vi "Para_ERD_Fxxx.vi"(7 "GEA Inputs":T4={"Source"=228, "Destination"=36} {"Destination" format="%.0x"; "Source" format="%.0x"}, 8 "Error In":errorcluster, 10 "Read ERD List":T2[](array[typedef])=[{"ERD Number"=62976, "Data Type"=enum."string"}, {"ERD Number"=62977, "Data Type"=enum."string"}, {"ERD Number"=63015, "Data Type"=enum."string"}, {"ERD Number"=63016, "Data Type"=enum."string"}, {"ERD Number"=63017, "Data Type"=enum."string"}, {"ERD Number"=63018, "Data Type"=enum."string"}, {"ERD Number"=63019, "Data Type"=enum."string"}, {"ERD Number"=63020, "Data Type"=enum."string"}, {"ERD Number"=63021, "Data Type"=enum."string"}, {"ERD Number"=63022, "Data Type"=enum."string"}, {"ERD Number"=63023, "Data Type"=enum."string"}, {"ERD Number"=63024, "Data Type"=enum."string"}, {"ERD Number"=63025, "Data Type"=enum."string"}, {"ERD Number"=63026, "Data Type"=enum."string"}, {"ERD Number"=63028, "Data Type"=enum."string"}, {"ERD Number"=63029, "Data Type"=enum."string"}, {"ERD Number"=63030, "Data Type"=enum."string"}, {"ERD Number"=63031, "Data Type"=enum."string"}, {"ERD Number"=63032, "Data Type"=enum."string"}, {"ERD Number"=63033, "Data Type"=enum."string"}, {"ERD Number"=63034, "Data Type"=enum."string"}, {"ERD Number"=63035, "Data Type"=enum."string"}, {"ERD Number"=63036, "Data Type"=enum."string"}, {"ERD Number"=63037, "Data Type"=enum."string"}, {"ERD Number"=63038, "Data Type"=enum."string"}, {"ERD Number"=63039, "Data Type"=enum."string"}, {"ERD Number"=63040, "Data Type"=enum."string"}, {"ERD Number"=63041, "Data Type"=enum."string"}, {"ERD Number"=63042, "Data Type"=enum."string"}, {"ERD Number"=63043, "Data Type"=enum."string"}, {"ERD Number"=63044, "Data Type"=enum."string"}, {"ERD Number"=63045, "Data Type"=enum."string"}, {"ERD Number"=63046, "Data Type"=enum."string"}, {"ERD Number"=63047, "Data Type"=enum."string"}, {"ERD Number"=63048, "Data Type"=enum."string"}, {"ERD Number"=63049, "Data Type"=enum."string"}, {"ERD Number"=63050, "Data Type"=enum."string"}, {"ERD Number"=63052, "Data Type"=enum."string"}, {"ERD Number"=63053, "Data Type"=enum."string"}, {"ERD Number"=63054, "Data Type"=enum."string"}, {"ERD Number"=63055, "Data Type"=enum."string"}, {"ERD Number"=63056, "Data Type"=enum."string"}, {"ERD Number"=63060, "Data Type"=enum."string"}, {"ERD Number"=63061, "Data Type"=enum."string"}, {"ERD Number"=63067, "Data Type"=enum."string"}, {"ERD Number"=63068, "Data Type"=enum."string"}, {"ERD Number"=63072, "Data Type"=enum."string"}, {"ERD Number"=63073, "Data Type"=enum."string"}, {"ERD Number"=63074, "Data Type"=enum."string"}, {"ERD Number"=63075, "Data Type"=enum."string"}, {"ERD Number"=63076, "Data Type"=enum."string"}, {"ERD Number"=63077, "Data Type"=enum."string"}, {"ERD Number"=63078, "Data Type"=enum."string"}, {"ERD Number"=63079, "Data Type"=enum."string"}, {"ERD Number"=63080, "Data Type"=enum."string"}, {"ERD Number"=63081, "Data Type"=enum."string"}] {"ERD Number" format="%.0x"}, 11 "GEA2 Reference In":refnum<k24>) -> (0 "Error Out":errorcluster, 1 "ERD Data Out":T3[](array[typedef]) {"ERD Number" format="%.0x"}, 2 "F6XX":T1, 3 "GEA2 Reference Out":refnum<k24>)   [LabVIEW 2023]
uses:
  type defs/F6_ERD_Control.ctl
  Common/LabVIEW GEA2 Toolkit/GEA3/type defs/Source_Destination.ctl
  D:/Common/LabVIEW GEA2 Toolkit/source/GEA3 DLL Source/GeaCommunication.dll
  Common/LabVIEW GEA2 Toolkit/source/GEA3 DLL Source/GeaCommunication.dll
  Common/LabVIEW GEA2 Toolkit/GEA3/type defs/ERD Read Data Out.ctl
  Common/LabVIEW GEA2 Toolkit/GEA3/type defs/ERD Read Data In.ctl
panel:
  out "number":u32
  in  "F6XX 2":T1
  in  "F6XX":T1
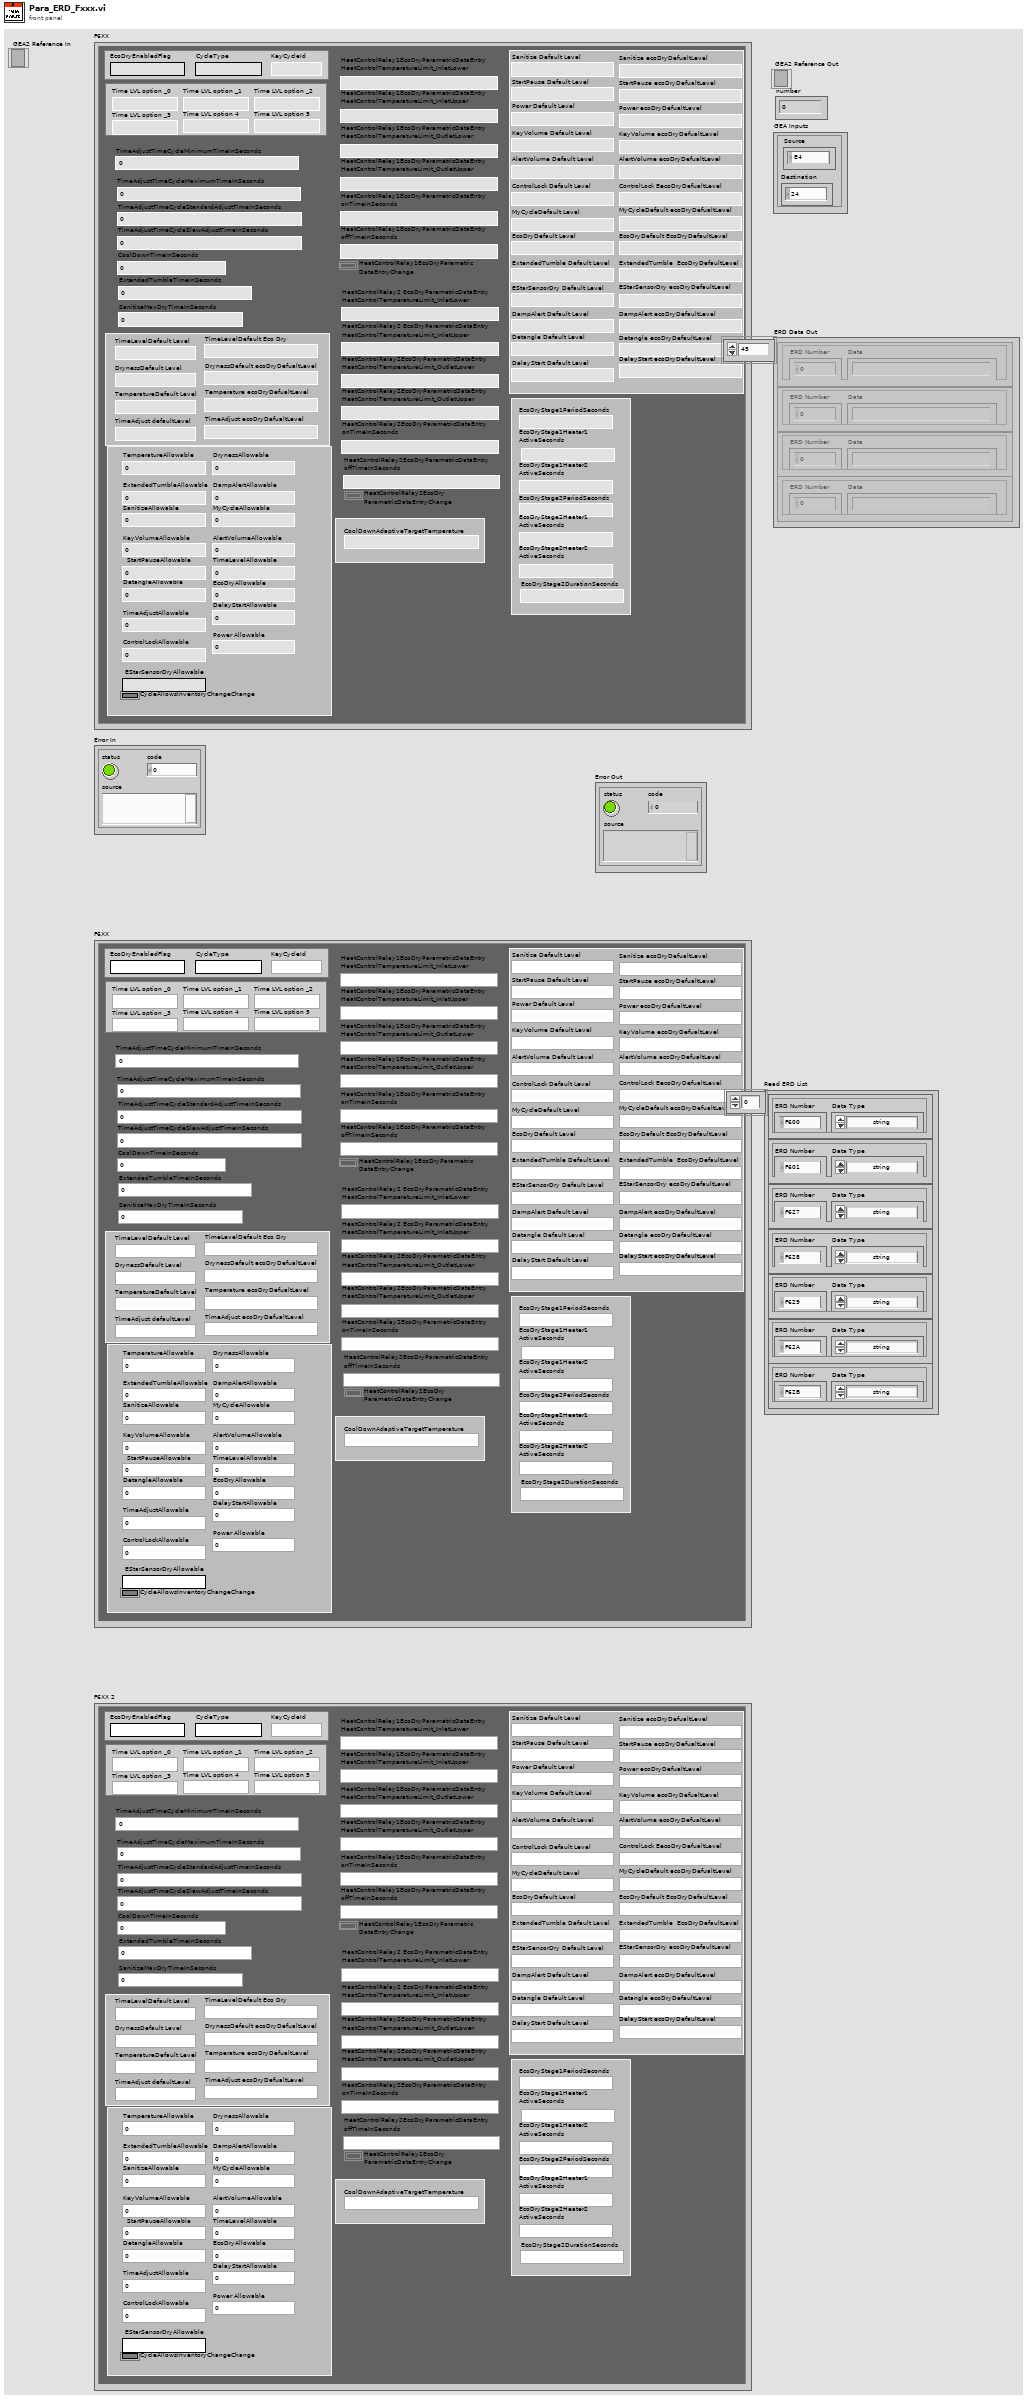
[diagram p1: front panel]
types:
  T1 = typedef "F6_ERD_Control.ctl" = cluster{"EcoDryEnabledFlag":string, "KeyCycleId":u8, "CycleType":string, "Time LVL option 5":u32, "Time LVL option 4":u32, "Time LVL option _3":u32, "Time LVL option _2":u32, "Time LVL option _1":u32, "Time LVL option _0":u32, "CoolDownTimeInSeconds":u32, "TimeAdjustTimeCycleMinimumTimeInSeconds":u32, "TimeAdjustTimeCycleMaximumTimeInSeconds":u32, "TimeAdjustTimeCycleStandardAdjustTimeInSeconds":u32, "TimeAdjustTimeCycleSlewAdjustTimeInSeconds":u32, "ExtendedTumbleTimeInSeconds":u32, "SanitizeMaxDryTimeInSeconds":u32, "TemperatureDefault Level":u8, "Temperature ecoDryDefualtLevel":u8, "DrynessDefault Level":u8, "DrynessDefault ecoDryDefualtLevel":u8, "TimeAdjust defaultLevel":u8, "TimeAdjust ecoDryDefualtLevel":u8, "TimeLevelDefault Level":u8, "TimeLevelDefault Eco Dry":u8, "EStarSensorDry Default Level":u8, "EStarSensorDry ecoDryDefaultLevel":u8, "EcoDryDefault Level":u8, "EcoDryDefault EcoDryDefaultLevel ":u8, "ExtendedTumble Default Level":u8, "ExtendedTumble  EcoDryDefaultLevel":u8, "Sanitize Default Level":u8, "Sanitize ecoDryDefualtLevel":u8, "MyCycleDefault Level":u8, "MyCycleDefault ecoDryDefualtLevel":u8, "StartPause Default Level":u8, "StartPause ecoDryDefualtLevel":u8, "Power Default Level":u8, "Power ecoDryDefualtLevel":u8, "KeyVolume Default Level":u8, "KeyVolume ecoDryDefualtLevel":u8, "AlertVolume Default Level":u8, "AlertVolume ecoDryDefualtLevel":u8, "ControlLock Default Level":u8, "ControlLock EecoDryDefualtLevel":u8, "HeatControlRelay1EcoDryParametricDataEntry\nHeatControlTemperatureLimit_InletLower":u16, "HeatControlRelay1EcoDryParametricDataEntry\nHeatControlTemperatureLimit_InletUpper":u16, "HeatControlRelay1EcoDryParametricDataEntry\nHeatControlTemperatureLimit_OutletLower":u16, "HeatControlRelay1EcoDryParametricDataEntry\nHeatControlTemperatureLimit_OutletUpper":u16, "HeatControlRelay1EcoDryParametricDataEntry\nonTimeInSeconds":u8, "HeatControlRelay1EcoDryParametricDataEntry\noffTimeInSeconds":u8, "HeatControlRelay1EcoDryParametric\nDataEntryChange ":bool, "HeatControlRelay2 EcoDryParametricDataEntry\nHeatControlTemperatureLimit_InletLower":u16, "HeatControlRelay2 EcoDryParametricDataEntry\nHeatControlTemperatureLimit_InletUpper ":u16, "HeatControlRelay2EcoDryParametricDataEntry\nHeatControlTemperatureLimit_OutletLower ":u16, "HeatControlRelay2EcoDryParametricDataEntry\nHeatControlTemperatureLimit_OutletUpper":u16, "HeatControlRelay2EcoDryParametricDataEntry\nonTimeInSeconds ":u8, "HeatControlRelay2EcoDryParametricDataEntry\noffTimeInSeconds ":u8, "HeatControlRelay2EcoDry\nParametricDataEntryChange":bool, "DampAlert Default Level":u8, "DampAlert ecoDryDefaultLevel":u8, "Detangle Default Level ":u8, "Detangle ecoDryDefaultLevel":u8, "DelayStart Default Level":u8, "DelayStart ecoDryDefaultLevel":u8, "CycleAllowsInventoryChangeChange":bool, "TemperatureAllowable":u8, "DrynessAllowable":u8, "TimeLevelAllowable":u8, "EcoDryAllowable":u8, "ExtendedTumbleAllowable":u8, "DampAlertAllowable":u8, "DetangleAllowable":u8, "DelayStartAllowable":u8, "SanitizeAllowable":u8, "MyCycleAllowable":u8, "TimeAdjustAllowable":u8, "Power Allowable":u8, "KeyVolumeAllowable":u8, "AlertVolumeAllowable":u8, "ControlLockAllowable":u8, "EStarSensorDryAllowable":string, "StartPauseAllowable":u8, "EcoDryStage1Heater2\nActiveSeconds":u32, "EcoDryStage2PeriodSeconds":u32, "EcoDryStage2Heater1\nActiveSeconds":u32, "EcoDryStage2Heater2\nActiveSeconds":u32, "EcoDryStage1Heater1\nActiveSeconds":u32, "EcoDryStage1PeriodSeconds":u32, "EcoDryStage2DurationSeconds":u32, "CoolDownAdaptiveTargetTemperature":u16}
  T2 = typedef "ERD Read Data In.ctl" = cluster{"ERD Number":u16, "Data Type":enum16{"string", "boolean", "uint8_t", "uint16_t", "uint32_t", "uint64_t", "int8_t", "int16_t", "int32_t", "int64_t"}}
  T3 = typedef "ERD Read Data Out.ctl" = cluster{"ERD Number":u16, "Data":string}
  T4 = typedef "Source_Destination.ctl" = cluster{"Source":u8, "Destination":u8}
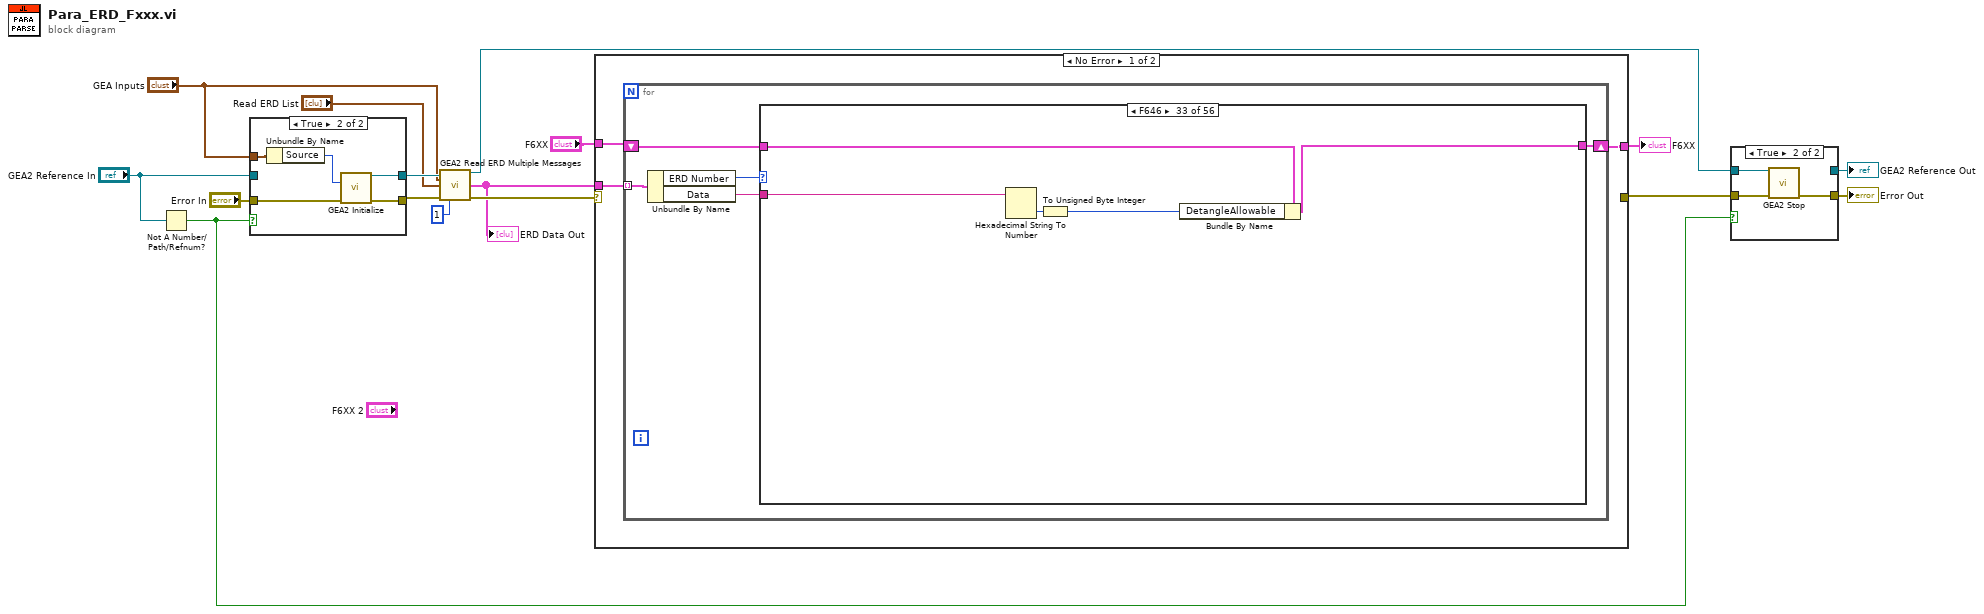
[diagram p0: block diagram]
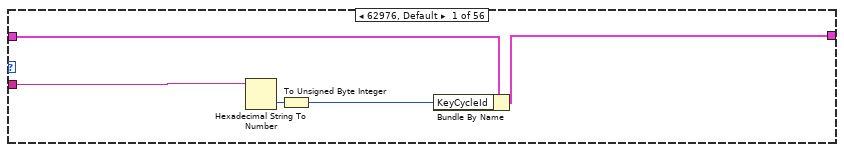
[diagram p4: hidden frame]
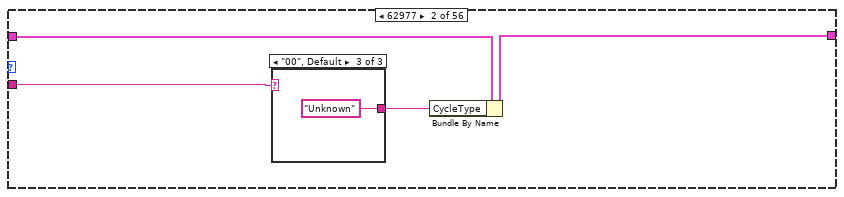
[diagram p5: hidden frame]
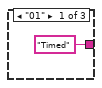
[diagram p6: hidden frame]
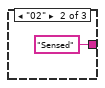
[diagram p7: hidden frame]
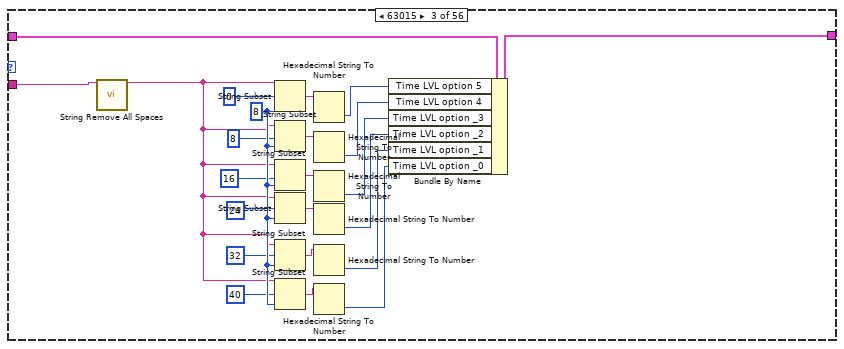
[diagram p8: hidden frame]
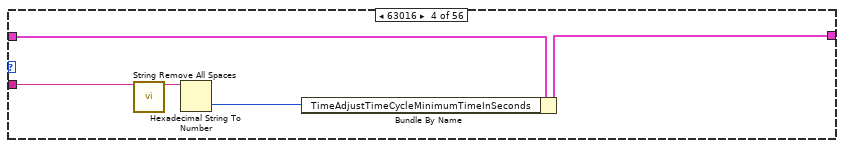
[diagram p9: hidden frame]
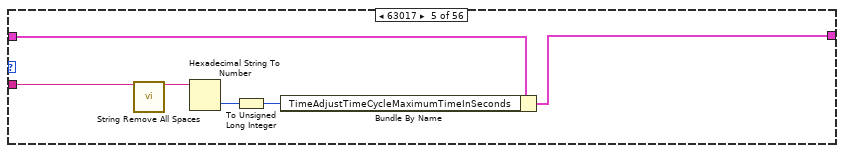
[diagram p10: hidden frame]
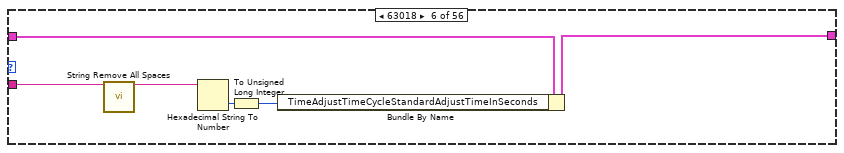
[diagram p11: hidden frame]
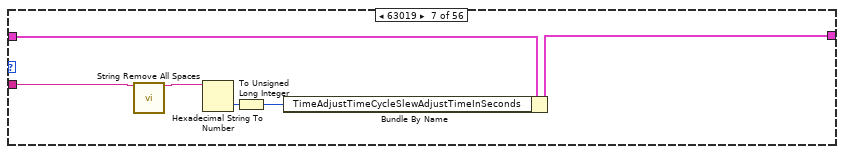
[diagram p12: hidden frame]
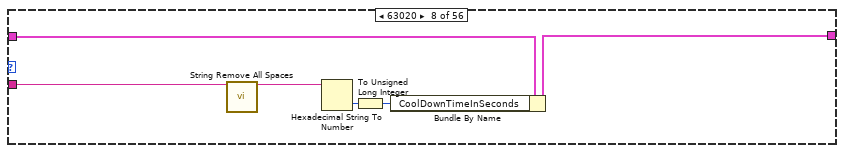
[diagram p13: hidden frame]
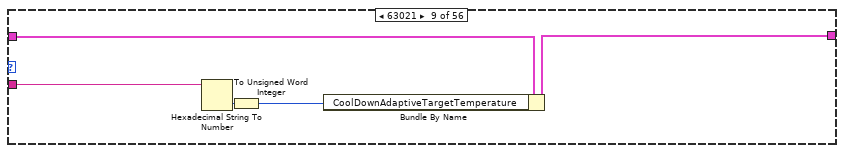
[diagram p14: hidden frame]
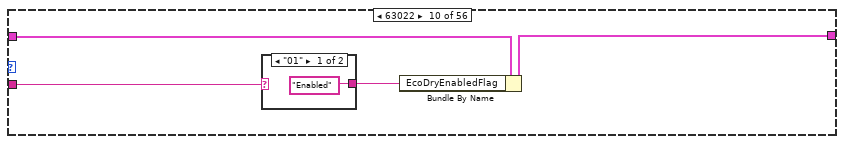
[diagram p15: hidden frame]
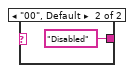
[diagram p16: hidden frame]
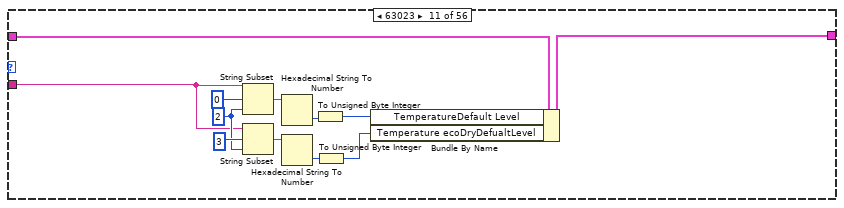
[diagram p17: hidden frame]
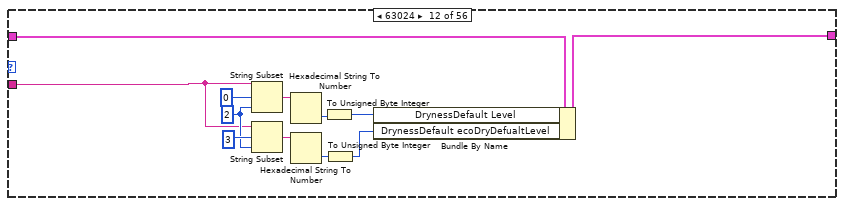
[diagram p18: hidden frame]
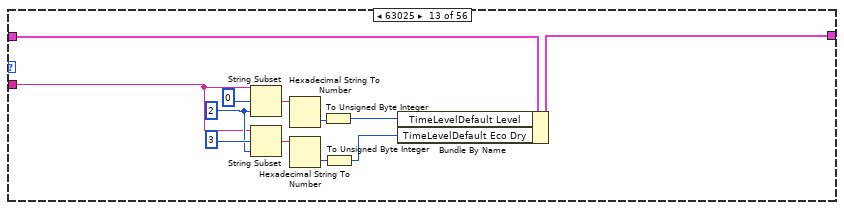
[diagram p19: hidden frame]
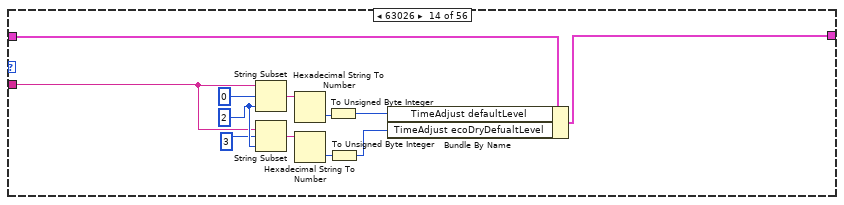
[diagram p20: hidden frame]
diagram:
  n1 = Not A Number/Path/Refnum?(number/path/refnum="GEA2 Reference In") -> (NaN/Path/Refnum?=w9:bool)
  n2 = case shown="True" w9 {
    tunnel: "Error In" -> [w17 w23]
    tunnel: [w17 w22] -> w13
    tunnel: "GEA2 Reference In" -> [w18 _]
    tunnel: [w18 w21] -> w11
    tunnel: "GEA Inputs" -> [_ w19]
    frame False {
    }
    frame True {
      n3 = Unbundle By Name(w19) -> ("Source"=w20:u8)
      n4 = call "GEA2 Initialize.vi"("Source Address"=w20, "error in"=w23) -> ("GEA2 Reference Out"=w21:refnum<k24>, "error out"=w22:errorcluster)  [unwired: 11 in, 1 out]
    }
  }
  n5 = call "GEA2 Read ERD Multiple Messages.vi"("GEA2 Reference In"=w11, "GEA Inputs"="GEA Inputs", "Read ERD List"="Read ERD List", "Error In"=w13, "#ERDs per message"=1) -> ("GEA2 Reference Out"=w7:refnum<k24>, "ERD Data Out"=w1:cluster{"ERD Number":u16, "Data":string}[], "Error Out"=w16:errorcluster)  [unwired: 7 in, 1 out]
  "ERD Data Out" <- w1
  n6 = case shown="No Error" w16 {
    selector: w16 -> [_ w522]
    tunnel: w1 -> [w26 _]
    tunnel: [w25 w523] -> w15
    tunnel: "F6XX" -> [w24 w523]
    tunnel: [_ w522] -> w6
    frame No Error {
      n7 = for {
        shift-right: [w30] -> w25
        shift-left: w24 -> [w31]
        tunnel: w26 -> [w28] mode=indexing
        n8 = Unbundle By Name(w28) -> ("ERD Number"=w29:u16, "Data"=w27:string)
        n9 = case shown="F646" w29 {
          tunnel: w31 -> [w35 w39 w66 w71 w75 w83 w89 w95 w100 w104 w118 w120 w133 w144 w156 w168 w181 w192 w204 w217 w229 w241 w253 w264 w277 w289 w303 w308 w313 w315 w320 w325 w331 w338 w340 w346 w351 w355 w361 w368 w373 w378 w382 w388 w390 w404 w440 w446 w480 w486 w489 w496 w501 w508 w514 w521]
          tunnel: [w36 w38 w65 w70 w76 w82 w88 w94 w99 w103 w117 w119 w132 w143 w155 w167 w180 w193 w205 w216 w228 w240 w252 w263 w276 w288 w302 w307 w312 w314 w321 w324 w330 w337 w339 w345 w350 w354 w360 w367 w372 w377 w381 w387 w389 w403 w439 w447 w479 w485 w490 w495 w502 w507 w513 w520] -> w30
          tunnel: w27 -> [w33 w40 w45 w69 w74 w79 w85 w91 w98 w102 w111 w121 w131 w145 w157 w169 w179 w191 w203 w215 w227 w239 w251 w265 w275 w287 w300 w305 w310 w316 w319 w326 w329 w334 w341 w344 w349 w356 w359 w365 w370 w375 w380 w384 w391 w402 w407 w442 w476 w482 w488 w493 w499 w506 w512 w519]
          frame 62976, Default {
            n10 = Hexadecimal String To Number(string=w33) -> (number=w34:u32)  [unwired: 2 in, 1 out]
            n11 = To Unsigned Byte Integer(number=w34) -> (unsigned 8bit integer=w32:u8)
            n12 = Bundle By Name(cluster=w35, "KeyCycleId"=w32) -> (w36:T1)
          }
          frame 62977 {
            n13 = case shown="\"00\", Default" w40 {
              tunnel: ["Timed" "Sensed" "Unknown"] -> w37
              frame "01" {
              }
              frame "02" {
              }
              frame "00", Default {
              }
            }
            n14 = Bundle By Name(cluster=w39, "CycleType"=w37) -> (w38:T1)
          }
          frame 63015 {
            w52 = 8 ("length (rest)")
            n15 = call "String Remove All Spaces.vi"("Input String"=w45) -> ("Spaces Removed"=w44:string)  [unwired: 13 in, 1 out]
            n16 = String Subset(string=w44, offset (0)=0, length (rest)=w52) -> (substring=w64:string)
            n17 = String Subset(string=w44, offset (0)=8, length (rest)=w52) -> (substring=w62:string)
            n18 = String Subset(string=w44, offset (0)=16, length (rest)=w52) -> (substring=w59:string)
            n19 = String Subset(string=w44, offset (0)=24, length (rest)=w52) -> (substring=w58:string)
            n20 = String Subset(string=w44, offset (0)=32, length (rest)=w52) -> (substring=w55:string)
            n21 = String Subset(string=w44, offset (0)=40, length (rest)=w52) -> (substring=w48:string)
            n22 = Hexadecimal String To Number(string=w64) -> (number=w60:u32)  [unwired: 2 in, 1 out]
            n23 = Hexadecimal String To Number(string=w62) -> (number=w61:u32)  [unwired: 2 in, 1 out]
            n24 = Hexadecimal String To Number(string=w59) -> (number=w57:u32)  [unwired: 2 in, 1 out]
            n25 = Hexadecimal String To Number(string=w58) -> (number=w56:u32)  [unwired: 2 in, 1 out]
            n26 = Hexadecimal String To Number(string=w55) -> (number=w54:u32)  [unwired: 2 in, 1 out]
            n27 = Hexadecimal String To Number(string=w48) -> (number=w53:u32)  [unwired: 2 in, 1 out]
            n28 = Bundle By Name(cluster=w66, "Time LVL option 5"=w60, "Time LVL option 4"=w61, "Time LVL option _3"=w57, "Time LVL option _2"=w56, "Time LVL option _1"=w54, "Time LVL option _0"=w53) -> (w65:T1)
          }
          frame 63016 {
            n29 = call "String Remove All Spaces.vi"("Input String"=w69) -> ("Spaces Removed"=w68:string)  [unwired: 13 in, 1 out]
            n30 = Hexadecimal String To Number(string=w68) -> (number=w67:u32)  [unwired: 2 in, 1 out]
            n31 = Bundle By Name(cluster=w71, "TimeAdjustTimeCycleMinimumTimeInSeconds"=w67) -> (w70:T1)
          }
          frame 63017 {
            n32 = call "String Remove All Spaces.vi"("Input String"=w74) -> ("Spaces Removed"=w73:string)  [unwired: 13 in, 1 out]
            n33 = Hexadecimal String To Number(string=w73) -> (number=w72:u32)  [unwired: 2 in, 1 out]
            n34 = To Unsigned Long Integer(number=w72) -> (unsigned 32bit integer=w77:u32)
            n35 = Bundle By Name(cluster=w75, "TimeAdjustTimeCycleMaximumTimeInSeconds"=w77) -> (w76:T1)
          }
          frame 63018 {
            n36 = call "String Remove All Spaces.vi"("Input String"=w79) -> ("Spaces Removed"=w78:string)  [unwired: 13 in, 1 out]
            n37 = Hexadecimal String To Number(string=w78) -> (number=w81:u32)  [unwired: 2 in, 1 out]
            n38 = To Unsigned Long Integer(number=w81) -> (unsigned 32bit integer=w80:u32)
            n39 = Bundle By Name(cluster=w83, "TimeAdjustTimeCycleStandardAdjustTimeInSeconds"=w80) -> (w82:T1)
          }
          frame 63019 {
            n40 = call "String Remove All Spaces.vi"("Input String"=w85) -> ("Spaces Removed"=w84:string)  [unwired: 13 in, 1 out]
            n41 = Hexadecimal String To Number(string=w84) -> (number=w87:u32)  [unwired: 2 in, 1 out]
            n42 = To Unsigned Long Integer(number=w87) -> (unsigned 32bit integer=w86:u32)
            n43 = Bundle By Name(cluster=w89, "TimeAdjustTimeCycleSlewAdjustTimeInSeconds"=w86) -> (w88:T1)
          }
          frame 63020 {
            n44 = call "String Remove All Spaces.vi"("Input String"=w91) -> ("Spaces Removed"=w90:string)  [unwired: 13 in, 1 out]
            n45 = Hexadecimal String To Number(string=w90) -> (number=w93:u32)  [unwired: 2 in, 1 out]
            n46 = To Unsigned Long Integer(number=w93) -> (unsigned 32bit integer=w92:u32)
            n47 = Bundle By Name(cluster=w95, "CoolDownTimeInSeconds"=w92) -> (w94:T1)
          }
          frame 63021 {
            n48 = Hexadecimal String To Number(string=w98) -> (number=w97:u32)  [unwired: 2 in, 1 out]
            n49 = To Unsigned Word Integer(number=w97) -> (unsigned 16bit integer=w96:u16)
            n50 = Bundle By Name(cluster=w100, "CoolDownAdaptiveTargetTemperature"=w96) -> (w99:T1)
          }
          frame 63022 {
            n51 = case shown="\"01\"" w102 {
              tunnel: ["Enabled" "Disabled"] -> w101
              frame "01" {
              }
              frame "00", Default {
              }
            }
            n52 = Bundle By Name(cluster=w104, "EcoDryEnabledFlag"=w101) -> (w103:T1)
          }
          frame 63023 {
            w112 = 2 ("length (rest)")
            n53 = String Subset(string=w111, offset (0)=0, length (rest)=w112) -> (substring=w116:string)
            n54 = String Subset(string=w111, offset (0)=3, length (rest)=w112) -> (substring=w113:string)
            n55 = Hexadecimal String To Number(string=w116) -> (number=w110:u32)  [unwired: 2 in, 1 out]
            n56 = Hexadecimal String To Number(string=w113) -> (number=w108:u32)  [unwired: 2 in, 1 out]
            n57 = To Unsigned Byte Integer(number=w110) -> (unsigned 8bit integer=w109:u8)
            n58 = To Unsigned Byte Integer(number=w108) -> (unsigned 8bit integer=w107:u8)
            n59 = Bundle By Name(cluster=w118, "TemperatureDefault Level"=w109, "Temperature ecoDryDefualtLevel"=w107) -> (w117:T1)
          }
          frame 63024 {
            w126 = 2 ("length (rest)")
            n60 = String Subset(string=w121, offset (0)=0, length (rest)=w126) -> (substring=w130:string)
            n61 = String Subset(string=w121, offset (0)=3, length (rest)=w126) -> (substring=w127:string)
            n62 = Hexadecimal String To Number(string=w130) -> (number=w125:u32)  [unwired: 2 in, 1 out]
            n63 = Hexadecimal String To Number(string=w127) -> (number=w123:u32)  [unwired: 2 in, 1 out]
            n64 = To Unsigned Byte Integer(number=w125) -> (unsigned 8bit integer=w124:u8)
            n65 = To Unsigned Byte Integer(number=w123) -> (unsigned 8bit integer=w122:u8)
            n66 = Bundle By Name(cluster=w120, "DrynessDefault Level"=w124, "DrynessDefault ecoDryDefualtLevel"=w122) -> (w119:T1)
          }
          frame 63025 {
            w138 = 2 ("length (rest)")
            n67 = String Subset(string=w131, offset (0)=0, length (rest)=w138) -> (substring=w142:string)
            n68 = String Subset(string=w131, offset (0)=3, length (rest)=w138) -> (substring=w139:string)
            n69 = Hexadecimal String To Number(string=w142) -> (number=w137:u32)  [unwired: 2 in, 1 out]
            n70 = Hexadecimal String To Number(string=w139) -> (number=w135:u32)  [unwired: 2 in, 1 out]
            n71 = To Unsigned Byte Integer(number=w137) -> (unsigned 8bit integer=w136:u8)
            n72 = To Unsigned Byte Integer(number=w135) -> (unsigned 8bit integer=w134:u8)
            n73 = Bundle By Name(cluster=w133, "TimeLevelDefault Level"=w136, "TimeLevelDefault Eco Dry"=w134) -> (w132:T1)
          }
          frame 63026 {
            w151 = 2 ("length (rest)")
            n74 = String Subset(string=w145, offset (0)=0, length (rest)=w151) -> (substring=w154:string)
            n75 = String Subset(string=w145, offset (0)=3, length (rest)=w151) -> (substring=w152:string)
            n76 = Hexadecimal String To Number(string=w154) -> (number=w150:u32)  [unwired: 2 in, 1 out]
            n77 = Hexadecimal String To Number(string=w152) -> (number=w148:u32)  [unwired: 2 in, 1 out]
            n78 = To Unsigned Byte Integer(number=w150) -> (unsigned 8bit integer=w149:u8)
            n79 = To Unsigned Byte Integer(number=w148) -> (unsigned 8bit integer=w147:u8)
            n80 = Bundle By Name(cluster=w144, "TimeAdjust defaultLevel"=w149, "TimeAdjust ecoDryDefualtLevel"=w147) -> (w143:T1)
          }
          frame 63028 {
            w163 = 2 ("length (rest)")
            n81 = String Subset(string=w157, offset (0)=0, length (rest)=w163) -> (substring=w166:string)
            n82 = String Subset(string=w157, offset (0)=3, length (rest)=w163) -> (substring=w164:string)
            n83 = Hexadecimal String To Number(string=w166) -> (number=w162:u32)  [unwired: 2 in, 1 out]
            n84 = Hexadecimal String To Number(string=w164) -> (number=w160:u32)  [unwired: 2 in, 1 out]
            n85 = To Unsigned Byte Integer(number=w162) -> (unsigned 8bit integer=w161:u8)
            n86 = To Unsigned Byte Integer(number=w160) -> (unsigned 8bit integer=w159:u8)
            n87 = Bundle By Name(cluster=w156, "EcoDryDefault Level"=w161, "EcoDryDefault EcoDryDefaultLevel"=w159) -> (w155:T1)
          }
          frame 63029 {
            w175 = 2 ("length (rest)")
            n88 = String Subset(string=w169, offset (0)=0, length (rest)=w175) -> (substring=w178:string)
            n89 = String Subset(string=w169, offset (0)=3, length (rest)=w175) -> (substring=w176:string)
            n90 = Hexadecimal String To Number(string=w178) -> (number=w174:u32)  [unwired: 2 in, 1 out]
            n91 = Hexadecimal String To Number(string=w176) -> (number=w172:u32)  [unwired: 2 in, 1 out]
            n92 = To Unsigned Byte Integer(number=w174) -> (unsigned 8bit integer=w173:u8)
            n93 = To Unsigned Byte Integer(number=w172) -> (unsigned 8bit integer=w171:u8)
            n94 = Bundle By Name(cluster=w168, "ExtendedTumble Default Level"=w173, "ExtendedTumble  EcoDryDefaultLevel"=w171) -> (w167:T1)
          }
          frame 63030 {
            w187 = 2 ("length (rest)")
            n95 = String Subset(string=w179, offset (0)=0, length (rest)=w187) -> (substring=w190:string)
            n96 = String Subset(string=w179, offset (0)=3, length (rest)=w187) -> (substring=w188:string)
            n97 = Hexadecimal String To Number(string=w190) -> (number=w186:u32)  [unwired: 2 in, 1 out]
            n98 = Hexadecimal String To Number(string=w188) -> (number=w184:u32)  [unwired: 2 in, 1 out]
            n99 = To Unsigned Byte Integer(number=w186) -> (unsigned 8bit integer=w185:u8)
            n100 = To Unsigned Byte Integer(number=w184) -> (unsigned 8bit integer=w183:u8)
            n101 = Bundle By Name(cluster=w181, "DampAlert Default Level"=w185, "DampAlert ecoDryDefaultLevel"=w183) -> (w180:T1)
          }
          frame 63031 {
            w199 = 2 ("length (rest)")
            n102 = String Subset(string=w191, offset (0)=0, length (rest)=w199) -> (substring=w202:string)
            n103 = String Subset(string=w191, offset (0)=3, length (rest)=w199) -> (substring=w200:string)
            n104 = Hexadecimal String To Number(string=w202) -> (number=w198:u32)  [unwired: 2 in, 1 out]
            n105 = Hexadecimal String To Number(string=w200) -> (number=w196:u32)  [unwired: 2 in, 1 out]
            n106 = To Unsigned Byte Integer(number=w198) -> (unsigned 8bit integer=w197:u8)
            n107 = To Unsigned Byte Integer(number=w196) -> (unsigned 8bit integer=w195:u8)
            n108 = Bundle By Name(cluster=w192, "Detangle Default Level"=w197, "Detangle ecoDryDefaultLevel"=w195) -> (w193:T1)
          }
          frame 63032 {
            w211 = 2 ("length (rest)")
            n109 = String Subset(string=w203, offset (0)=0, length (rest)=w211) -> (substring=w214:string)
            n110 = String Subset(string=w203, offset (0)=3, length (rest)=w211) -> (substring=w212:string)
            n111 = Hexadecimal String To Number(string=w214) -> (number=w210:u32)  [unwired: 2 in, 1 out]
            n112 = Hexadecimal String To Number(string=w212) -> (number=w208:u32)  [unwired: 2 in, 1 out]
            n113 = To Unsigned Byte Integer(number=w210) -> (unsigned 8bit integer=w209:u8)
            n114 = To Unsigned Byte Integer(number=w208) -> (unsigned 8bit integer=w207:u8)
            n115 = Bundle By Name(cluster=w204, "DelayStart Default Level"=w209, "DelayStart ecoDryDefaultLevel"=w207) -> (w205:T1)
          }
          frame 63033 {
            w223 = 2 ("length (rest)")
            n116 = String Subset(string=w215, offset (0)=0, length (rest)=w223) -> (substring=w226:string)
            n117 = String Subset(string=w215, offset (0)=3, length (rest)=w223) -> (substring=w224:string)
            n118 = Hexadecimal String To Number(string=w226) -> (number=w222:u32)  [unwired: 2 in, 1 out]
            n119 = Hexadecimal String To Number(string=w224) -> (number=w220:u32)  [unwired: 2 in, 1 out]
            n120 = To Unsigned Byte Integer(number=w222) -> (unsigned 8bit integer=w221:u8)
            n121 = To Unsigned Byte Integer(number=w220) -> (unsigned 8bit integer=w219:u8)
            n122 = Bundle By Name(cluster=w217, "Sanitize Default Level"=w221, "Sanitize ecoDryDefualtLevel"=w219) -> (w216:T1)
          }
          frame 63034 {
            w235 = 2 ("length (rest)")
            n123 = String Subset(string=w227, offset (0)=0, length (rest)=w235) -> (substring=w238:string)
            n124 = String Subset(string=w227, offset (0)=3, length (rest)=w235) -> (substring=w236:string)
            n125 = Hexadecimal String To Number(string=w238) -> (number=w234:u32)  [unwired: 2 in, 1 out]
            n126 = Hexadecimal String To Number(string=w236) -> (number=w232:u32)  [unwired: 2 in, 1 out]
            n127 = To Unsigned Byte Integer(number=w234) -> (unsigned 8bit integer=w233:u8)
            n128 = To Unsigned Byte Integer(number=w232) -> (unsigned 8bit integer=w231:u8)
            n129 = Bundle By Name(cluster=w229, "MyCycleDefault Level"=w233, "MyCycleDefault ecoDryDefualtLevel"=w231) -> (w228:T1)
          }
          frame 63035 {
            w247 = 2 ("length (rest)")
            n130 = String Subset(string=w239, offset (0)=0, length (rest)=w247) -> (substring=w250:string)
            n131 = String Subset(string=w239, offset (0)=3, length (rest)=w247) -> (substring=w248:string)
            n132 = Hexadecimal String To Number(string=w250) -> (number=w246:u32)  [unwired: 2 in, 1 out]
            n133 = Hexadecimal String To Number(string=w248) -> (number=w244:u32)  [unwired: 2 in, 1 out]
            n134 = To Unsigned Byte Integer(number=w246) -> (unsigned 8bit integer=w245:u8)
            n135 = To Unsigned Byte Integer(number=w244) -> (unsigned 8bit integer=w243:u8)
            n136 = Bundle By Name(cluster=w241, "StartPause Default Level"=w245, "StartPause ecoDryDefualtLevel"=w243) -> (w240:T1)
          }
          frame 63036 {
            w259 = 2 ("length (rest)")
            n137 = String Subset(string=w251, offset (0)=0, length (rest)=w259) -> (substring=w262:string)
            n138 = String Subset(string=w251, offset (0)=3, length (rest)=w259) -> (substring=w260:string)
            n139 = Hexadecimal String To Number(string=w262) -> (number=w258:u32)  [unwired: 2 in, 1 out]
            n140 = Hexadecimal String To Number(string=w260) -> (number=w256:u32)  [unwired: 2 in, 1 out]
            n141 = To Unsigned Byte Integer(number=w258) -> (unsigned 8bit integer=w257:u8)
            n142 = To Unsigned Byte Integer(number=w256) -> (unsigned 8bit integer=w255:u8)
            n143 = Bundle By Name(cluster=w253, "Power Default Level"=w257, "Power ecoDryDefualtLevel"=w255) -> (w252:T1)
          }
          frame 63037 {
            w271 = 2 ("length (rest)")
            n144 = String Subset(string=w265, offset (0)=0, length (rest)=w271) -> (substring=w274:string)
            n145 = String Subset(string=w265, offset (0)=3, length (rest)=w271) -> (substring=w272:string)
            n146 = Hexadecimal String To Number(string=w274) -> (number=w270:u32)  [unwired: 2 in, 1 out]
            n147 = Hexadecimal String To Number(string=w272) -> (number=w268:u32)  [unwired: 2 in, 1 out]
            n148 = To Unsigned Byte Integer(number=w270) -> (unsigned 8bit integer=w269:u8)
            n149 = To Unsigned Byte Integer(number=w268) -> (unsigned 8bit integer=w267:u8)
            n150 = Bundle By Name(cluster=w264, "KeyVolume Default Level"=w269, "KeyVolume ecoDryDefualtLevel"=w267) -> (w263:T1)
          }
          frame 63038 {
            w281 = 2 ("length (rest)")
            n151 = String Subset(string=w275, offset (0)=0, length (rest)=w281) -> (substring=w278:string)
            n152 = String Subset(string=w275, offset (0)=3, length (rest)=w281) -> (substring=w280:string)
            n153 = Hexadecimal String To Number(string=w278) -> (number=w282:u32)  [unwired: 2 in, 1 out]
            n154 = Hexadecimal String To Number(string=w280) -> (number=w284:u32)  [unwired: 2 in, 1 out]
            n155 = To Unsigned Byte Integer(number=w282) -> (unsigned 8bit integer=w283:u8)
            n156 = To Unsigned Byte Integer(number=w284) -> (unsigned 8bit integer=w285:u8)
            n157 = Bundle By Name(cluster=w277, "AlertVolume Default Level"=w283, "AlertVolume ecoDryDefualtLevel"=w285) -> (w276:T1)
          }
          frame 63039 {
            w295 = 2 ("length (rest)")
            n158 = String Subset(string=w287, offset (0)=0, length (rest)=w295) -> (substring=w298:string)
            n159 = String Subset(string=w287, offset (0)=3, length (rest)=w295) -> (substring=w296:string)
            n160 = Hexadecimal String To Number(string=w298) -> (number=w294:u32)  [unwired: 2 in, 1 out]
            n161 = Hexadecimal String To Number(string=w296) -> (number=w292:u32)  [unwired: 2 in, 1 out]
            n162 = To Unsigned Byte Integer(number=w294) -> (unsigned 8bit integer=w293:u8)
            n163 = To Unsigned Byte Integer(number=w292) -> (unsigned 8bit integer=w291:u8)
            n164 = Bundle By Name(cluster=w289, "ControlLock Default Level"=w293, "ControlLock EecoDryDefualtLevel"=w291) -> (w288:T1)
          }
          frame 63040 {
            n165 = Hexadecimal String To Number(string=w300) -> (number=w301:u32)  [unwired: 2 in, 1 out]
            n166 = To Unsigned Byte Integer(number=w301) -> (unsigned 8bit integer=w299:u8)
            n167 = Bundle By Name(cluster=w303, "TemperatureAllowable"=w299) -> (w302:T1)
          }
          frame 63041 {
            n168 = Hexadecimal String To Number(string=w305) -> (number=w306:u32)  [unwired: 2 in, 1 out]
            n169 = To Unsigned Byte Integer(number=w306) -> (unsigned 8bit integer=w304:u8)
            n170 = Bundle By Name(cluster=w308, "DrynessAllowable"=w304) -> (w307:T1)
          }
          frame 63042 {
            n171 = Hexadecimal String To Number(string=w310) -> (number=w311:u32)  [unwired: 2 in, 1 out]
            n172 = To Unsigned Byte Integer(number=w311) -> (unsigned 8bit integer=w309:u8)
            n173 = Bundle By Name(cluster=w313, "TimeLevelAllowable"=w309) -> (w312:T1)
          }
          frame 63043 {
            n174 = Hexadecimal String To Number(string=w316) -> (number=w318:u32)  [unwired: 2 in, 1 out]
            n175 = To Unsigned Byte Integer(number=w318) -> (unsigned 8bit integer=w317:u8)
            n176 = Bundle By Name(cluster=w315, "EcoDryAllowable"=w317) -> (w314:T1)
          }
          frame 63044 {
            n177 = Hexadecimal String To Number(string=w319) -> (number=w323:u32)  [unwired: 2 in, 1 out]
            n178 = To Unsigned Byte Integer(number=w323) -> (unsigned 8bit integer=w322:u8)
            n179 = Bundle By Name(cluster=w320, "ExtendedTumbleAllowable"=w322) -> (w321:T1)
          }
          frame 63045 {
            n180 = Hexadecimal String To Number(string=w326) -> (number=w328:u32)  [unwired: 2 in, 1 out]
            n181 = To Unsigned Byte Integer(number=w328) -> (unsigned 8bit integer=w327:u8)
            n182 = Bundle By Name(cluster=w325, "DampAlertAllowable"=w327) -> (w324:T1)
          }
          frame 63046 {
            n183 = Hexadecimal String To Number(string=w329) -> (number=w333:u32)  [unwired: 2 in, 1 out]
            n184 = To Unsigned Byte Integer(number=w333) -> (unsigned 8bit integer=w332:u8)
            n185 = Bundle By Name(cluster=w331, "DetangleAllowable"=w332) -> (w330:T1)
          }
          frame 63047 {
            n186 = Hexadecimal String To Number(string=w334) -> (number=w336:u32)  [unwired: 2 in, 1 out]
            n187 = To Unsigned Byte Integer(number=w336) -> (unsigned 8bit integer=w335:u8)
            n188 = Bundle By Name(cluster=w338, "DelayStartAllowable"=w335) -> (w337:T1)
          }
          frame 63048 {
            n189 = Hexadecimal String To Number(string=w341) -> (number=w343:u32)  [unwired: 2 in, 1 out]
            n190 = To Unsigned Byte Integer(number=w343) -> (unsigned 8bit integer=w342:u8)
            n191 = Bundle By Name(cluster=w340, "SanitizeAllowable"=w342) -> (w339:T1)
          }
          frame 63049 {
            n192 = Hexadecimal String To Number(string=w344) -> (number=w348:u32)  [unwired: 2 in, 1 out]
            n193 = To Unsigned Byte Integer(number=w348) -> (unsigned 8bit integer=w347:u8)
            n194 = Bundle By Name(cluster=w346, "MyCycleAllowable"=w347) -> (w345:T1)
          }
          frame 63050 {
            n195 = Hexadecimal String To Number(string=w349) -> (number=w353:u32)  [unwired: 2 in, 1 out]
            n196 = To Unsigned Byte Integer(number=w353) -> (unsigned 8bit integer=w352:u8)
            n197 = Bundle By Name(cluster=w351, "TimeLevelAllowable"=w352) -> (w350:T1)
          }
          frame 63052 {
            n198 = Hexadecimal String To Number(string=w356) -> (number=w358:u32)  [unwired: 2 in, 1 out]
            n199 = To Unsigned Byte Integer(number=w358) -> (unsigned 8bit integer=w357:u8)
            n200 = Bundle By Name(cluster=w355, "StartPauseAllowable"=w357) -> (w354:T1)
          }
          frame 63053 {
            n201 = Hexadecimal String To Number(string=w359) -> (number=w363:u32)  [unwired: 2 in, 1 out]
            n202 = To Unsigned Byte Integer(number=w363) -> (unsigned 8bit integer=w362:u8)
            n203 = Bundle By Name(cluster=w361, "Power Allowable"=w362) -> (w360:T1)
          }
          frame 63054 {
            n204 = Hexadecimal String To Number(string=w365) -> (number=w366:u32)  [unwired: 2 in, 1 out]
            n205 = To Unsigned Byte Integer(number=w366) -> (unsigned 8bit integer=w364:u8)
            n206 = Bundle By Name(cluster=w368, "KeyVolumeAllowable"=w364) -> (w367:T1)
          }
          frame 63055 {
            n207 = Hexadecimal String To Number(string=w370) -> (number=w371:u32)  [unwired: 2 in, 1 out]
            n208 = To Unsigned Byte Integer(number=w371) -> (unsigned 8bit integer=w369:u8)
            n209 = Bundle By Name(cluster=w373, "AlertVolumeAllowable"=w369) -> (w372:T1)
          }
          frame 63056 {
            n210 = Hexadecimal String To Number(string=w375) -> (number=w376:u32)  [unwired: 2 in, 1 out]
            n211 = To Unsigned Byte Integer(number=w376) -> (unsigned 8bit integer=w374:u8)
            n212 = Bundle By Name(cluster=w378, "ControlLockAllowable"=w374) -> (w377:T1)
          }
          frame 63060 {
            n213 = call "HexStringToBoolean.vi"("Hex String"=w380) -> ("Boolean"=w379:bool)
            n214 = Bundle By Name(cluster=w382, "CycleAllowsInventoryChangeChange"=w379) -> (w381:T1)
          }
          frame 63061 {
            n215 = call "String Remove All Spaces.vi"("Input String"=w384) -> ("Spaces Removed"=w383:string)  [unwired: 13 in, 1 out]
            n216 = Decimal String To Number(string=w383) -> (number=w386:i32)  [unwired: 2 in, 1 out]
            n217 = To Unsigned Long Integer(number=w386) -> (unsigned 32bit integer=w385:u32)
            n218 = Bundle By Name(cluster=w388, "ExtendedTumbleTimeInSeconds"=w385) -> (w387:T1)
          }
          frame 63067 {
            w395 = 2 ("length (rest)")
            n219 = String Subset(string=w391, offset (0)=0, length (rest)=w395) -> (substring=w392:string)
            n220 = String Subset(string=w391, offset (0)=3, length (rest)=w395) -> (substring=w394:string)
            n221 = Hexadecimal String To Number(string=w392) -> (number=w396:u32)  [unwired: 2 in, 1 out]
            n222 = Hexadecimal String To Number(string=w394) -> (number=w398:u32)  [unwired: 2 in, 1 out]
            n223 = To Unsigned Byte Integer(number=w396) -> (unsigned 8bit integer=w397:u8)
            n224 = To Unsigned Byte Integer(number=w398) -> (unsigned 8bit integer=w399:u8)
            n225 = Bundle By Name(cluster=w390, "EStarSensorDry Default Level"=w397, "EStarSensorDry ecoDryDefaultLevel"=w399) -> (w389:T1)
          }
          frame 63068 {
            n226 = case shown="\"01,02,03\"" w402 {
              tunnel: ["Enabled" "Disabled"] -> w401
              frame "01,02,03" {
              }
              frame "00", Default {
              }
            }
            n227 = Bundle By Name(cluster=w404, "EStarSensorDryAllowable"=w401) -> (w403:T1)
          }
          frame 63072 {
            w411 = 2 ("length (rest)")
            w413 = 4 ("length (rest)")
            n228 = call "String Remove All Spaces.vi"("Input String"=w407) -> ("Spaces Removed"=w408:string)  [unwired: 13 in, 1 out]
            n229 = String Subset(string=w408, offset (0)=0, length (rest)=w413) -> (substring=w438:string)
            n230 = String Subset(string=w408, offset (0)=4, length (rest)=w413) -> (substring=w436:string)
            n231 = String Subset(string=w408, offset (0)=8, length (rest)=w413) -> (substring=w435:string)
            n232 = String Subset(string=w408, offset (0)=12, length (rest)=w413) -> (substring=w434:string)
            n233 = String Subset(string=w408, offset (0)=16, length (rest)=w411) -> (substring=w433:string)
            n234 = String Subset(string=w408, offset (0)=18, length (rest)=w411) -> (substring=w415:string)
            n235 = String Subset(string=w408, offset (0)=20, length (rest)=w411) -> (substring=w410:string)
            n236 = Hexadecimal String To Number(string=w438) -> (number=w427:u32)  [unwired: 2 in, 1 out]
            n237 = Hexadecimal String To Number(string=w436) -> (number=w425:u32)  [unwired: 2 in, 1 out]
            n238 = Hexadecimal String To Number(string=w435) -> (number=w423:u32)  [unwired: 2 in, 1 out]
            n239 = Hexadecimal String To Number(string=w434) -> (number=w421:u32)  [unwired: 2 in, 1 out]
            n240 = Hexadecimal String To Number(string=w433) -> (number=w418:u32)  [unwired: 2 in, 1 out]
            n241 = Hexadecimal String To Number(string=w415) -> (number=w419:u32)  [unwired: 2 in, 1 out]
            n242 = call "String Remove All Spaces.vi"("Input String"=w410) -> ("Spaces Removed"=w409:string)  [unwired: 13 in, 1 out]
            n243 = To Unsigned Word Integer(number=w427) -> (unsigned 16bit integer=w426:u16)
            n244 = To Unsigned Word Integer(number=w425) -> (unsigned 16bit integer=w424:u16)
            n245 = To Unsigned Word Integer(number=w423) -> (unsigned 16bit integer=w422:u16)
            n246 = To Unsigned Word Integer(number=w421) -> (unsigned 16bit integer=w420:u16)
            n247 = To Unsigned Byte Integer(number=w418) -> (unsigned 8bit integer=w417:u8)
            n248 = To Unsigned Byte Integer(number=w419) -> (unsigned 8bit integer=w416:u8)
            n249 = call "HexStringToBoolean.vi"("Hex String"=w409) -> ("Boolean"=w412:bool)
            n250 = Bundle By Name(cluster=w440, "HeatControlRelay1EcoDryParametricDataEntry\nHeatControlTemperatureLimit_InletLower"=w426, "HeatControlRelay1EcoDryParametricDataEntry\nHeatControlTemperatureLimit_InletUpper"=w424, "HeatControlRelay1EcoDryParametricDataEntry\nHeatControlTemperatureLimit_OutletLower"=w422, "HeatControlRelay1EcoDryParametricDataEntry\nHeatControlTemperatureLimit_OutletUpper"=w420, "HeatControlRelay1EcoDryParametricDataEntry\nonTimeInSeconds"=w417, "HeatControlRelay1EcoDryParametricDataEntry\noffTimeInSeconds"=w416, "HeatControlRelay1EcoDryParametric\nDataEntryChange"=w412) -> (w439:T1)
          }
          frame 63073 {
            w445 = 2 ("length (rest)")
            w448 = 4 ("length (rest)")
            n251 = call "String Remove All Spaces.vi"("Input String"=w442) -> ("Spaces Removed"=w441:string)  [unwired: 13 in, 1 out]
            n252 = String Subset(string=w441, offset (0)=0, length (rest)=w448) -> (substring=w474:string)
            n253 = String Subset(string=w441, offset (0)=4, length (rest)=w448) -> (substring=w472:string)
            n254 = String Subset(string=w441, offset (0)=8, length (rest)=w448) -> (substring=w471:string)
            n255 = String Subset(string=w441, offset (0)=12, length (rest)=w448) -> (substring=w470:string)
            n256 = String Subset(string=w441, offset (0)=16, length (rest)=w445) -> (substring=w469:string)
            n257 = String Subset(string=w441, offset (0)=18, length (rest)=w445) -> (substring=w451:string)
            n258 = String Subset(string=w441, offset (0)=20, length (rest)=w445) -> (substring=w444:string)
            n259 = Hexadecimal String To Number(string=w474) -> (number=w463:u32)  [unwired: 2 in, 1 out]
            n260 = Hexadecimal String To Number(string=w472) -> (number=w461:u32)  [unwired: 2 in, 1 out]
            n261 = Hexadecimal String To Number(string=w471) -> (number=w459:u32)  [unwired: 2 in, 1 out]
            n262 = Hexadecimal String To Number(string=w470) -> (number=w457:u32)  [unwired: 2 in, 1 out]
            n263 = Hexadecimal String To Number(string=w469) -> (number=w454:u32)  [unwired: 2 in, 1 out]
            n264 = Hexadecimal String To Number(string=w451) -> (number=w455:u32)  [unwired: 2 in, 1 out]
            n265 = call "String Remove All Spaces.vi"("Input String"=w444) -> ("Spaces Removed"=w443:string)  [unwired: 13 in, 1 out]
            n266 = To Unsigned Word Integer(number=w463) -> (unsigned 16bit integer=w462:u16)
            n267 = To Unsigned Word Integer(number=w461) -> (unsigned 16bit integer=w460:u16)
            n268 = To Unsigned Word Integer(number=w459) -> (unsigned 16bit integer=w458:u16)
            n269 = To Unsigned Word Integer(number=w457) -> (unsigned 16bit integer=w456:u16)
            n270 = To Unsigned Byte Integer(number=w454) -> (unsigned 8bit integer=w453:u8)
            n271 = To Unsigned Byte Integer(number=w455) -> (unsigned 8bit integer=w452:u8)
            n272 = call "HexStringToBoolean.vi"("Hex String"=w443) -> ("Boolean"=w449:bool)
            n273 = Bundle By Name(cluster=w446, "HeatControlRelay2 EcoDryParametricDataEntry\nHeatControlTemperatureLimit_InletLower"=w462, "HeatControlRelay2 EcoDryParametricDataEntry\nHeatControlTemperatureLimit_InletUpper"=w460, "HeatControlRelay2EcoDryParametricDataEntry\nHeatControlTemperatureLimit_OutletLower"=w458, "HeatControlRelay2EcoDryParametricDataEntry\nHeatControlTemperatureLimit_OutletUpper"=w456, "HeatControlRelay2EcoDryParametricDataEntry\nonTimeInSeconds"=w453, "HeatControlRelay2EcoDryParametricDataEntry\noffTimeInSeconds"=w452, "HeatControlRelay2EcoDry\nParametricDataEntryChange"=w449) -> (w447:T1)
          }
          frame 63074 {
            n274 = call "String Remove All Spaces.vi"("Input String"=w476) -> ("Spaces Removed"=w475:string)  [unwired: 13 in, 1 out]
            n275 = Hexadecimal String To Number(string=w475) -> (number=w478:u32)  [unwired: 2 in, 1 out]
            n276 = To Unsigned Long Integer(number=w478) -> (unsigned 32bit integer=w477:u32)
            n277 = Bundle By Name(cluster=w480, "EcoDryStage2DurationSeconds"=w477) -> (w479:T1)
          }
          frame 63075 {
            n278 = call "String Remove All Spaces.vi"("Input String"=w482) -> ("Spaces Removed"=w481:string)  [unwired: 13 in, 1 out]
            n279 = Hexadecimal String To Number(string=w481) -> (number=w484:u32)  [unwired: 2 in, 1 out]
            n280 = To Unsigned Long Integer(number=w484) -> (unsigned 32bit integer=w483:u32)
            n281 = Bundle By Name(cluster=w486, "EcoDryStage1PeriodSeconds"=w483) -> (w485:T1)
          }
          frame 63076 {
            n282 = call "String Remove All Spaces.vi"("Input String"=w488) -> ("Spaces Removed"=w487:string)  [unwired: 13 in, 1 out]
            n283 = Hexadecimal String To Number(string=w487) -> (number=w492:u32)  [unwired: 2 in, 1 out]
            n284 = To Unsigned Long Integer(number=w492) -> (unsigned 32bit integer=w491:u32)
            n285 = Bundle By Name(cluster=w489, "EcoDryStage1Heater1\nActiveSeconds"=w491) -> (w490:T1)
          }
          frame 63077 {
            n286 = call "String Remove All Spaces.vi"("Input String"=w493) -> ("Spaces Removed"=w494:string)  [unwired: 13 in, 1 out]
            n287 = Hexadecimal String To Number(string=w494) -> (number=w498:u32)  [unwired: 2 in, 1 out]
            n288 = To Unsigned Long Integer(number=w498) -> (unsigned 32bit integer=w497:u32)
            n289 = Bundle By Name(cluster=w496, "EcoDryStage1Heater2\nActiveSeconds"=w497) -> (w495:T1)
          }
          frame 63078 {
            n290 = call "String Remove All Spaces.vi"("Input String"=w499) -> ("Spaces Removed"=w500:string)  [unwired: 13 in, 1 out]
            n291 = Hexadecimal String To Number(string=w500) -> (number=w504:u32)  [unwired: 2 in, 1 out]
            n292 = To Unsigned Long Integer(number=w504) -> (unsigned 32bit integer=w503:u32)
            n293 = Bundle By Name(cluster=w501, "EcoDryStage2PeriodSeconds"=w503) -> (w502:T1)
          }
          frame 63079 {
            n294 = call "String Remove All Spaces.vi"("Input String"=w506) -> ("Spaces Removed"=w505:string)  [unwired: 13 in, 1 out]
            n295 = Hexadecimal String To Number(string=w505) -> (number=w510:u32)  [unwired: 2 in, 1 out]
            n296 = To Unsigned Long Integer(number=w510) -> (unsigned 32bit integer=w509:u32)
            n297 = Bundle By Name(cluster=w508, "EcoDryStage2Heater1\nActiveSeconds"=w509) -> (w507:T1)
          }
          frame 63080 {
            n298 = call "String Remove All Spaces.vi"("Input String"=w512) -> ("Spaces Removed"=w511:string)  [unwired: 13 in, 1 out]
            n299 = Hexadecimal String To Number(string=w511) -> (number=w516:u32)  [unwired: 2 in, 1 out]
            n300 = To Unsigned Long Integer(number=w516) -> (unsigned 32bit integer=w515:u32)
            n301 = Bundle By Name(cluster=w514, "EcoDryStage2Heater2\nActiveSeconds"=w515) -> (w513:T1)
          }
          frame 63081 {
            n302 = call "String Remove All Spaces.vi"("Input String"=w519) -> ("Spaces Removed"=w518:string)  [unwired: 13 in, 1 out]
            n303 = Hexadecimal String To Number(string=w518) -> (number=w517:u32)  [unwired: 2 in, 1 out]
            "number" <- w517
            n304 = Bundle By Name(cluster=w521, "SanitizeMaxDryTimeInSeconds"=w517) -> (w520:T1)
          }
        }
      }
    }
    frame Error {
    }
  }
  "F6XX" <- w15
  n305 = case shown="True" w9 {
    tunnel: [w524 w528] -> w8
    tunnel: w7 -> [w525 w527]
    tunnel: [w525 _] -> w5
    tunnel: w6 -> [w524 w526]
    frame False {
    }
    frame True {
      n306 = call "GEA2 Stop.vi"("GEA2 Reference In"=w527, "Error In"=w526) -> ("Error Out"=w528:errorcluster)  [unwired: 13 in]
    }
  }
  "Error Out" <- w8
  "GEA2 Reference Out" <- w5
